vi "Display Info.vi"(7 "Layout ref":refnum<vi>, 8 "error in (no error)":errorcluster, 9 "Modify (F) /Add [T]":bool, 10 "Names in use":string[](array[string])=["PB", "Feet"], 11 "Slave_Line in":refnum<class "Slave_Line.lvclass">) -> (0 "error out":errorcluster, 1 "Names in use out":string[](array[string]), 2 "Changes Made?":bool, 3 "Slave_Line out":refnum<class "Slave_Line.lvclass">)   [LabVIEW 2013, in "Slave_Line.lvclass"]
uses:
  Slave_Line.lvclass
  TypeDefs/DigitalColumnAppearCluster.ctl
  Slave_Line.lvclass/Slave_Line.ctl
  ColumnVIs/Column/Column.lvclass
panel:
  in  "Master Channel":i32
  in  "Slave Column":T1={"Column Name"="", "Width"=15, "Bkgd"=[1985280, 6618880, 14090026], "Text"=[16448250, 0, 0]}
  in  "Name":string="Feet"
  in  "Device Description":string="Othe rfeet"
  in  "Cancel":bool
  in  "Done":bool
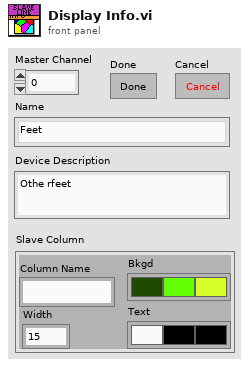
[diagram p1: front panel]
types:
  T1 = typedef "DigitalColumnAppearCluster.ctl" = cluster{"Column Name":string, "Width":u32, "Bkgd":u32[], "Text":u32[]}
  T2 = typedef "ColumnAppearCluster.ctl" = cluster{"Column Name":string, "Width":u32, "Bkgd":u32[], "Text":u32[]}
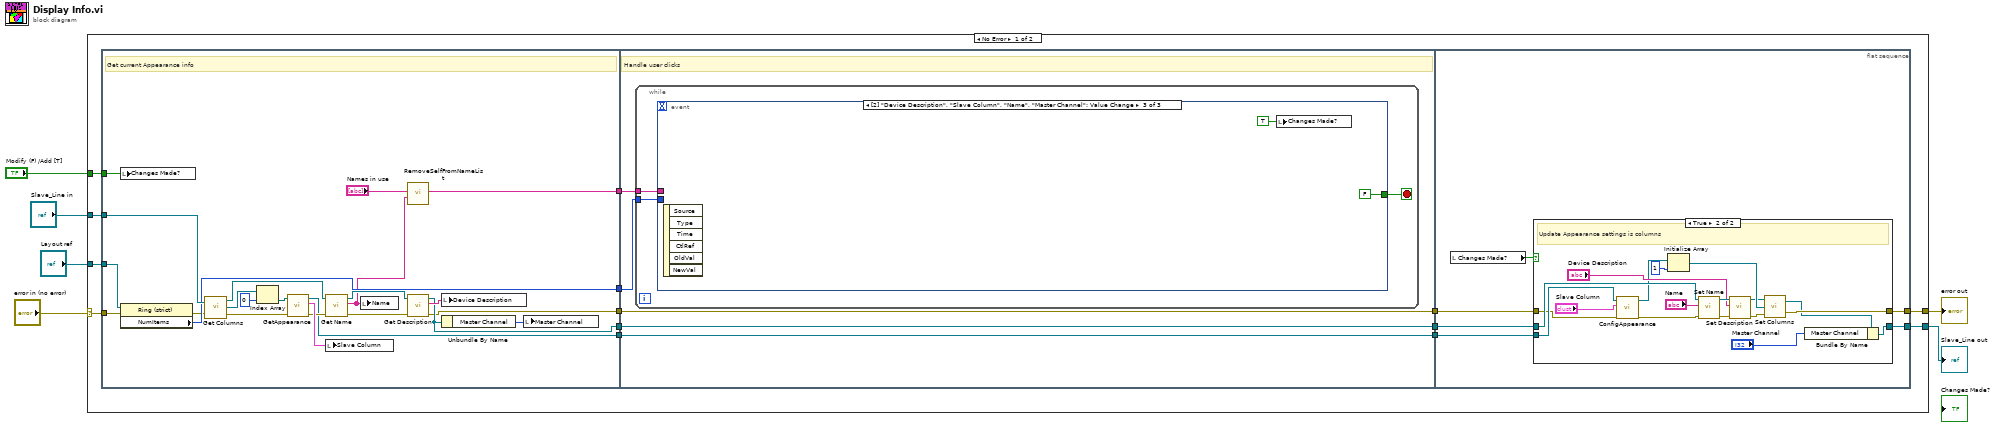
[diagram p0: block diagram]
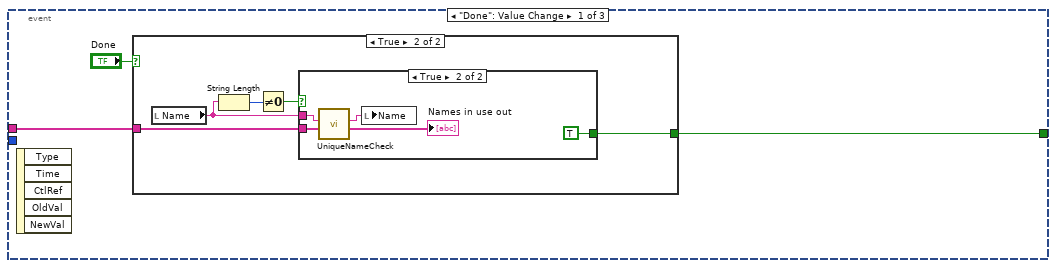
[diagram p2: hidden frame]
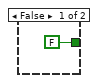
[diagram p3: hidden frame]
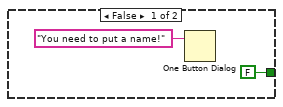
[diagram p4: hidden frame]
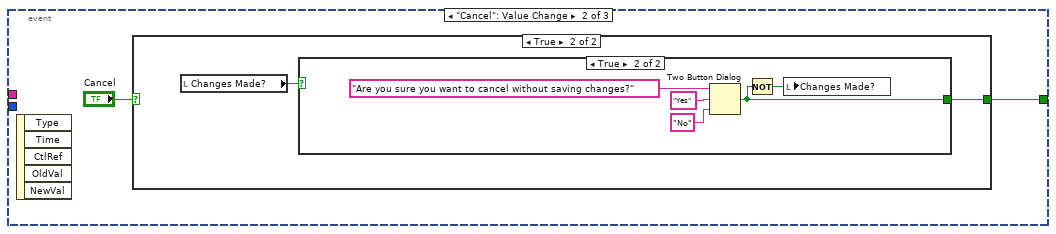
[diagram p5: hidden frame]
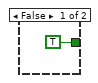
[diagram p7: hidden frame]
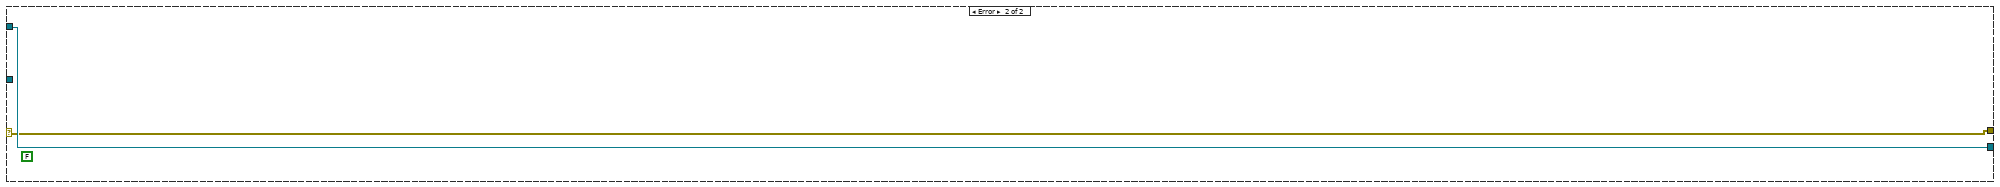
[diagram p9: hidden frame]
diagram:
  n1 = case shown="No Error" "error in (no error)" {
    selector: "error in (no error)" -> [w13 w107]
    tunnel: [w15 w108] -> w2
    tunnel: "Slave_Line in" -> [w20 w108]
    tunnel: [w14 w107] -> w1
    tunnel: "Layout ref" -> [w12 _]
    tunnel: "Modify (F) /Add [T]" -> [w10 _]
    frame No Error {
      n2 = flat-sequence {
        tunnel: w20 -> [w41]
        tunnel: [w27] -> w19
        tunnel: [w26] -> w17
        tunnel: w13 -> [w37]
        tunnel: w12 -> [w38]
        tunnel: [w36] -> w11
        tunnel: w10 -> [w35]
        tunnel: [w32] -> w9
        tunnel: [w22] -> w8
        tunnel: w19 -> [w48]
        tunnel: [w48] -> w18
        tunnel: w17 -> [w47]
        tunnel: [w47] -> w16
        tunnel: w11 -> [w46]
        tunnel: w9 -> [w45]
        tunnel: w8 -> [w44]
        tunnel: [w44] -> w7
        tunnel: w18 -> [w85]
        tunnel: w16 -> [w82]
        tunnel: [w84] -> w15
        tunnel: [w83] -> w14
        tunnel: w7 -> [w81]
        frame #0 {
          # "Get current Appearance info"
          n3 = local write "Changes Made?"(w35) -> ()
          n4 = property class="Ring (strict)"(reference=w38, error in=w37) -> (error out=w24:errorcluster, "NumItems"=w36:u32)  [unwired: 1 out]
          n5 = call-dynamic "Get Columns.vi"("Device in"=w41, "error in (no error)"=w24) -> ("Device out"=w39:refnum<class "Slave_Line.lvclass">, "Columns"=w31:refnum<class "Column.lvclass">[], "error out"=w25:errorcluster)
          n6 = Index Array(array=w31, index=0) -> (element=w29:refnum<class "Column.lvclass">)
          n7 = call "GetAppearance.vi"("error in (no error)"=w25, "Column in"=w29) -> ("error out"=w23:errorcluster, "Column Appearance"=w28:T2, "Column out"=w22:refnum<class "Column.lvclass">)  [unwired: 7 in]
          n8 = call-dynamic "Get Name.vi"("error in (no error)"=w23, "Device in"=w39) -> ("error out"=w40:errorcluster, "Name"=w33:string, "Device out"=w43:refnum<class "Slave_Line.lvclass">)  [unwired: 7 in]
          n9 = local write "Slave Column"(w28) -> ()
          n10 = local write "Name"(w33) -> ()
          n11 = call "RemoveSelfFromNameList.vi"("self Name"=w33, "Names in use"="Names in use") -> ("Reserved Names"=w32:string[])  [unwired: 9 in]
          n12 = call-dynamic "Get Description.vi"("error in (no error)"=w40, "Device in"=w43) -> ("error out"=w26:errorcluster, "Device Description"=w42:string, "Device out"=w27:refnum<class "Slave_Line.lvclass">)  [unwired: 7 in]
          n13 = local write "Device Description"(w42) -> ()
          n14 = Unbundle By Name(w27) -> ("Master Channel"=w21:i32)
          n15 = local write "Master Channel"(w21) -> ()
        }
        frame #1 {
          # "Handle user clicks"
          n16 = while {
            tunnel: w46 -> [w50]
            tunnel: w45 -> [w49]
            stop <- w51 stop-if-true
            n17 = event shown="[2] \"Device Description\", \"Slave Column\", \"Name\", \"Master Channel\": Value Change" {
              selector: _ -> [_ _ _]
              dyn-events: _ -> [_ _ _]
              timeout: _ -> [_ _ _]
              tunnel: [w53 w69 FALSE ("T button?")] -> w51
              tunnel: w50 -> [_ _ _]
              tunnel: w49 -> [w52 _ _]
              event "Done": Value Change {
                n18 = event-data() -> ()  [unwired: 1 in, 5 out]
                n19 = case shown="True" "Done" {
                  tunnel: [FALSE w58] -> w53
                  tunnel: w52 -> [_ w56]
                  frame False {
                  }
                  frame True {
                    n20 = local read "Name"() -> (w57:string)
                    n21 = String Length(string=w57) -> (length=w60:i32)
                    n22 = Not Equal To 0?(x=w60) -> (x != 0?=w59:bool)
                    n23 = case shown="True" w59 {
                      tunnel: [FALSE TRUE] -> w58
                      tunnel: w57 -> [_ w66]
                      tunnel: w56 -> [_ w64]
                      frame False {
                        n24 = One Button Dialog(message="You need to put a name!") -> ()  [unwired: 1 in, 1 out]
                      }
                      frame True {
                        n25 = call "UniqueNameCheck.vi"("Names in use"=w64, "Device Name"=w66) -> ("Names in use out"=→"Names in use out":string[], "Unique name"=w65:string)  [unwired: 8 in]
                        n26 = local write "Name"(w65) -> ()
                      }
                    }
                  }
                }
              }
              event "Cancel": Value Change {
                n27 = event-data() -> ()  [unwired: 1 in, 5 out]
                n28 = case shown="True" "Cancel" {
                  selector: "Cancel" -> [w70 _]
                  tunnel: [w70 w72] -> w69
                  frame False {
                  }
                  frame True {
                    n29 = local read "Changes Made?"() -> (w71:bool)
                    n30 = case shown="True" w71 {
                      tunnel: [TRUE w75] -> w72
                      frame False {
                      }
                      frame True {
                        n31 = Two Button Dialog(message="Are you sure you want to cancel without saving changes?", 1:"No", 2:"Yes") -> (T button?=w75:bool)
                        n32 = Not(x=w75) -> (.not. x?=w74:bool)
                        n33 = local write "Changes Made?"(w74) -> ()
                      }
                    }
                  }
                }
              }
              event "Device Description", "Name", "Master Channel": Value Change {
                n34 = event-data() -> ()  [unwired: 1 in, 6 out]
                n35 = local write "Changes Made?"(TRUE) -> ()
              }
            }
          }
        }
        frame #2 {
          n36 = local read "Changes Made?"() -> (w86:bool)
          n37 = case shown="True" w86 {
            tunnel: w85 -> [w88 w102]
            tunnel: [w87 w100] -> w83
            tunnel: [w88 w89] -> w84
            tunnel: w82 -> [w87 w94]
            tunnel: w81 -> [_ w98]
            frame False {
            }
            frame True {
              # "Update Appearance settings is columns"
              n38 = call "ConfigAppearance.vi"("error in (no error)"=w94, "Column Appearance"="Slave Column", "Column in"=w98) -> ("error out"=w93:errorcluster, "Column out"=w97:refnum<class "Column.lvclass">)  [unwired: 7 in]
              n39 = Initialize Array(w97, 1 ("dimension size")) -> (w95:refnum<class "Column.lvclass">[])
              n40 = call-dynamic "Set Name.vi"("error in (no error)"=w93, "Name"="Name", "Device in"=w102) -> ("error out"=w106:errorcluster, "Device out"=w105:refnum<class "Slave_Line.lvclass">)  [unwired: 7 in]
              n41 = call-dynamic "Set Description.vi"("error in (no error)"=w106, "Device Description"="Device Description", "Device in"=w105) -> ("error out"=w101:errorcluster, "Device out"=w92:refnum<class "Slave_Line.lvclass">)  [unwired: 7 in]
              n42 = call-dynamic "Set Columns.vi"("error in (no error)"=w101, "Columns"=w95, "Device in"=w92) -> ("error out"=w100:errorcluster, "Device out"=w90:refnum<class "Slave_Line.lvclass">)  [unwired: 1 in]
              n43 = Bundle By Name(cluster=w90, "Master Channel"="Master Channel") -> (w89:refnum<class "Slave_Line.lvclass">)
            }
          }
        }
      }
    }
    frame Error {
      (unwired) FALSE
    }
  }
  "error out" <- w1
  "Slave_Line out" <- w2
